vi "Power User.vi"(8 "PowerUser":enum16{"Check user", "Read status"}(ring), 11 "User Information":T1 caption="Informacion del usario" {"Country" items=["Afghanistan", "Aland Islands", "Albania", "Algeria", "American Samoa", "Andorra", "Angola", "Anguilla", "Antarctica", "Antigua And Barbuda", "Argentina", "Armenia", "Aruba", "Australia", "Austria", "Azerbaijan", "Bahamas", "Bahrain", "Bangladesh", "Barbados", "Belarus", "Belgium", "Belize", "Benin", "Bermuda", "Bhutan", "Bolivia", "Bosnia And Herzegovina", "Botswana", "Bouvet Island", "Brazil", "British Indian Ocean Territory", "Brunei Darussalam", "Bulgaria", "Burkina Faso", "Burundi", "Cambodia", "Cameroon", "Canada", "Cape Verde", "Cayman Islands", "Central African Republic", "Chad", "Chile", "China", "Christmas Island", "Cocos (Keeling) Islands", "Colombia", "Comoros", "Congo", "Congo, The Democratic Republic Of The", "Cook Islands", "Costa Rica", "Cote D'Ivoire", "Croatia", "Cuba", "Cyprus", "Czech Republic", "Denmark", "Djibouti", "Dominica", "Dominican Republic", "Ecuador", "Egypt", "El Salvador", "Equatorial Guinea", "Eritrea", "Estonia", "Ethiopia", "Falkland Islands (Malvinas)", "Faroe Islands", "Fiji", "Finland", "France", "French Guiana", "French Polynesia", "French Southern Territories", "Gabon", "Gambia", "Georgia", "Germany", "Ghana", "Gibraltar", "Greece", "Greenland", "Grenada", "Guadeloupe", "Guam", "Guatemala", "Guernsey", "Guinea", "Guinea-Bissau", "Guyana", "Haiti", "Heard Island And Mcdonald Islands", "Holy See (Vatican City State)", "Honduras", "Hong Kong", "Hungary", "Iceland", "India", "Indonesia", "Iran, Islamic Republic Of", "Iraq", "Ireland", "Isle Of Man", "Israel", "Italy", "Jamaica", "Japan", "Jersey", "Jordan", "Kazakhstan", "Kenya", "Kiribati", "Korea, Democratic People'S Republic Of", "Korea, Republic Of", "Kuwait", "Kyrgyzstan", "Lao People'S Democratic Republic", "Latvia", "Lebanon", "Lesotho", "Liberia", "Libyan Arab Jamahiriya", "Liechtenstein", "Lithuania", "Luxembourg", "Macao", "Macedonia, The Former Yugoslav Republic Of", "Madagascar", "Malawi", "Malaysia", "Maldives", "Mali", "Malta", "Marshall Islands", "Martinique", "Mauritania", "Mauritius", "Mayotte", "Mexico", "Micronesia, Federated States Of", "Moldova, Republic Of", "Monaco", "Mongolia", "Montserrat", "Morocco", "Mozambique", "Myanmar", "Namibia", "Nauru", "Nepal", "Netherlands", "Netherlands Antilles", "New Caledonia", "New Zealand", "Nicaragua", "Niger", "Nigeria", "Niue", "Norfolk Island", "Northern Mariana Islands", "Norway", "Oman", "Pakistan", "Palau", "Palestinian Territory, Occupied", "Panama", "Papua New Guinea", "Paraguay", "Peru", "Philippines", "Pitcairn", "Poland", "Portugal", "Puerto Rico", "Qatar", "Reunion", "Romania", "Russian Federation", "Rwanda", "Saint Helena", "Saint Kitts And Nevis", "Saint Lucia", "Saint Pierre And Miquelon", "Saint Vincent And The Grenadines", "Samoa", "San Marino", "Sao Tome And Principe", "Saudi Arabia", "Senegal", "Serbia And Montenegro", "Seychelles", "Sierra Leone", "Singapore", "Slovakia", "Slovenia", "Solomon Islands", "Somalia", "South Africa", "South Georgia And The South Sandwich Islands", "Spain", "Sri Lanka", "Sudan", "Suriname", "Svalbard And Jan Mayen", "Swaziland", "Sweden", "Switzerland", "Syrian Arab Republic", "Taiwan, Province Of China", "Tajikistan", "Tanzania, United Republic Of", "Thailand", "Timor-Leste", "Togo", "Tokelau", "Tonga", "Trinidad And Tobago", "Tunisia", "Turkey", "Turkmenistan", "Turks And Caicos Islands", "Tuvalu", "Uganda", "Ukraine", "United Arab Emirates", "United Kingdom", "United States", "United States Minor Outlying Islands", "Uruguay", "Uzbekistan", "Vanuatu", "Venezuela", "Viet Nam", "Virgin Islands, British", "Virgin Islands, U.S.", "Wallis And Futuna", "Western Sahara", "Yemen", "Zambia", "Zimbabwe", "(Not Specified)"]}) -> (2 "Power User":bool, 3 "Cornell User":bool)   [LabVIEW 2015]
uses:
  User Information.ctl
  Country Ring.ctl
  AguaClara Library.lvlib
panel:
  out "result string":string
  in  "Super Power Users":string[](array[string])=["hmr6", "mw24"]
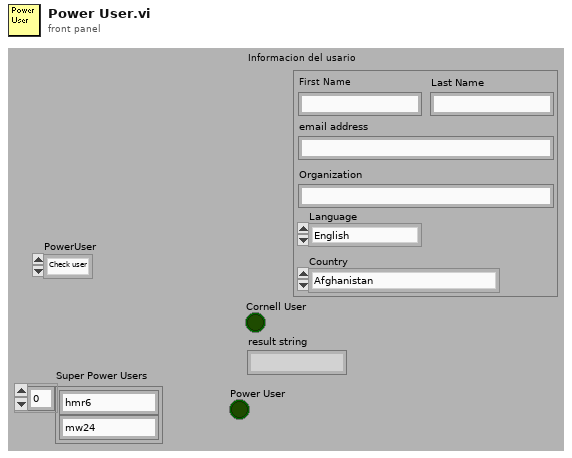
[diagram p1: front panel]
types:
  T1 = typedef "AguaClara Library.lvlib/User Information.ctl" = cluster{"First Name":string, "Last Name":string, "Email Address":string, "Organization":string, "Language":enum16{"English", "Español", "French"}, "Country":T2}
  T2 = typedef "Country Ring.ctl" = u16
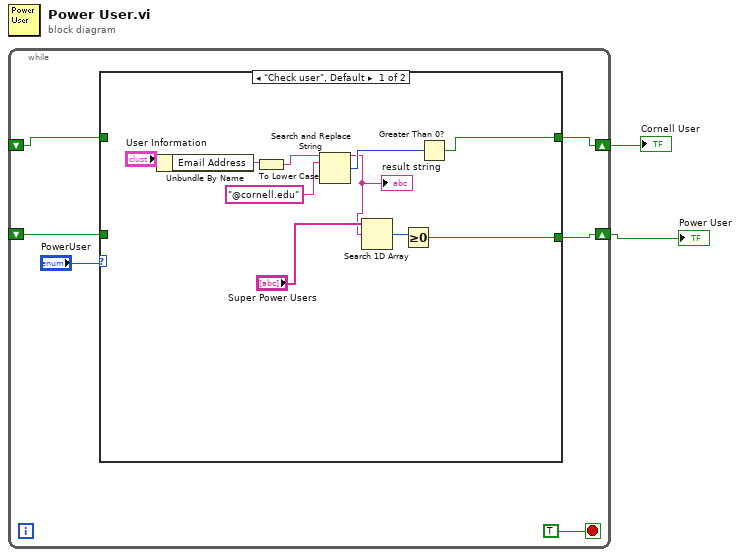
[diagram p0: block diagram]
diagram:
  n1 = while {
    shift-right: [w7] -> w2
    shift-left: _ -> [w5]
    shift-right: [w6] -> w1
    shift-left: _ -> [w4]
    stop <- TRUE stop-if-true
    n2 = case shown="\"Check user\", Default" "PowerUser" {
      tunnel: [w10 w20] -> w7
      tunnel: [w9 w19] -> w6
      tunnel: w5 -> [_ w20]
      tunnel: w4 -> [_ w19]
      frame "Check user", Default {
        n3 = Unbundle By Name("User Information") -> ("Email Address"=w17:string)
        n4 = To Lower Case(string=w17) -> (all lower case string=w15:string)
        n5 = Search and Replace String(input string=w15, search string="@cornell.edu") -> (result string=w12:string, number of replacements=w14:i32)  [unwired: 6 in, 2 out]
        "result string" <- w12
        n6 = Search 1D Array(1D array="Super Power Users", element=w12) -> (index of element=w11:i32)  [unwired: 1 in]
        n7 = Greater Or Equal To 0?(x=w11) -> (x >= 0?=w9:bool)
        n8 = Greater Than 0?(x=w14) -> (x > 0?=w10:bool)
      }
      frame "Read status" {
      }
    }
  }
  "Cornell User" <- w2
  "Power User" <- w1
